vi "com_read_ip.vi"() -> ()   [LabVIEW 2014]
panel:
  out "Indicator":bool
  in  "stop 2":bool
  # "BOMET TEST COMUNICATION READ"
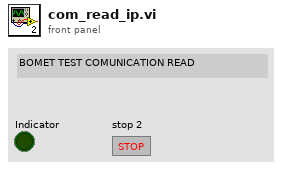
[diagram p1: front panel]
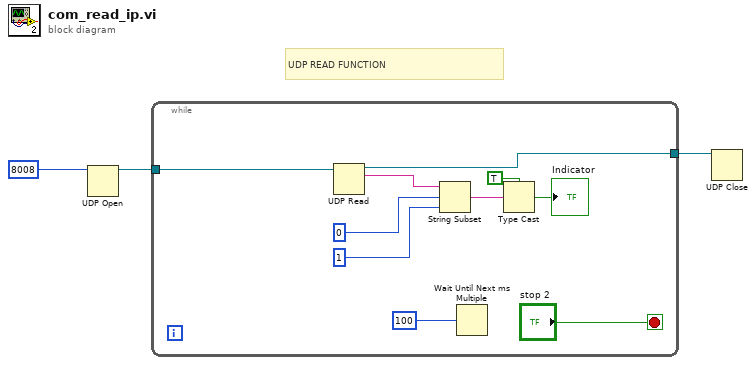
[diagram p0: block diagram]
diagram:
  # "UDP READ FUNCTION"
  n1 = UDP Open(11:u16 8008 ("port")) -> (port=w3:refnum<k16>)  [unwired: 4 in, 2 out]
  n2 = while {
    tunnel: w3 -> [w4]
    tunnel: [w13] -> w2
    stop <- "stop 2" stop-if-true
    n3 = UDP Read(connection ID=w4) -> (data out=w12:string, 3:w13:refnum<k16>)  [unwired: 3 in, 3 out]
    n4 = String Subset(string=w12, offset (0)=0, length (rest)=1 ("offset (0)")) -> (substring=w8:string)
    n5 = Wait Until Next ms Multiple(millisecond multiple=u32 100) -> ()  [unwired: 1 out]
    n6 = Type Cast(type=TRUE, x=w8) -> (*(type *) &x=→"Indicator":bool)
  }
  n7 = UDP Close(connection ID=w2) -> ()  [unwired: 1 in, 2 out]
